vi "IMU State Machine.vi"(0 "error in":errorcluster, 11 "IMU Command":T1) -> (2 "Gyro xyz (rad/s)":dbl[](array[numeric]), 3 "Acceleration x,y,z":dbl[](array[numeric]), 8 "error out":errorcluster)   [LabVIEW 2016]
uses:
  IMU Cmd.ctl
panel:
  out "Gyro x,y,z (deg/s)":dbl[](array[numeric])
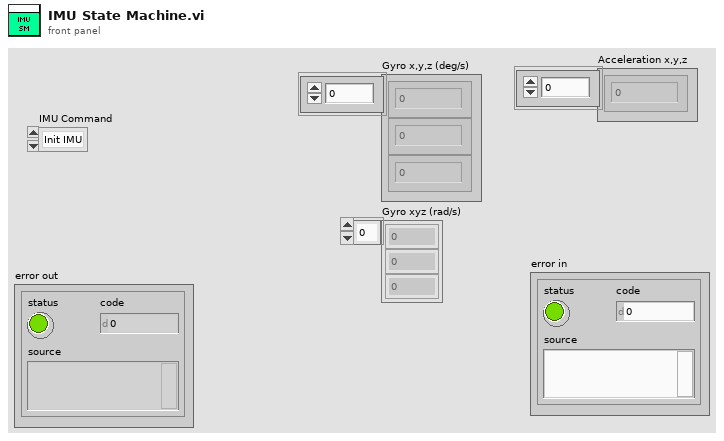
[diagram p1: front panel]
types:
  T1 = typedef "IMU Cmd.ctl" = enum16{"Init IMU", "Calibrate", "Read motion"}
  T2 = typedef "I2C.lvlib/I2C Reference.ctl" = cluster{"myRIO Reference":T3, "I2C Channels Enum":T7, "I2C Configuration":T8}
  T3 = typedef "myRIO Generic Hardware Reference.ctl" = cluster{"myRIO Model":T4, "myRIO Hardware Reference":T5}
  T4 = typedef "Hardware Version Enum.ctl" = enum16{"Unknown", "myRIO-1900", "myRIO-1950", "roboRIO", "NI ELVIS RIO CM"}
  T5 = typedef "myRIO v1.0 Reference.ctl" = cluster{"Generic FPGA Reference":T6, "Allow multiple opens":bool}
  T6 = typedef "Generic FPGA Reference.ctl" = refnum<k20>
  T7 = typedef "I2C Channels Enum.ctl" = enum16{"Not Connected", "A/I2C", "B/I2C", "I2C/I2C"}
  T8 = typedef "I2C.lvlib/I2C Configuration.ctl" = cluster{"I2C Transfer Rate":T9}
  T9 = typedef "I2C.lvlib/I2C Transfer Rate.ctl" = enum16{"Standard mode (100 kbps)", "Fast mode (400 kbps)"}
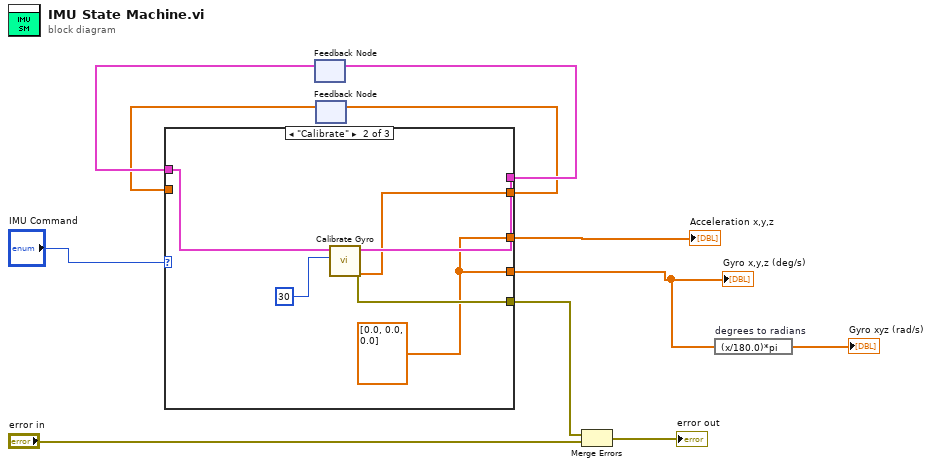
[diagram p0: block diagram]
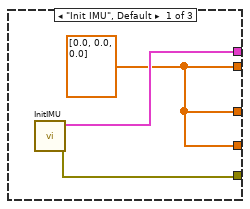
[diagram p2: hidden frame]
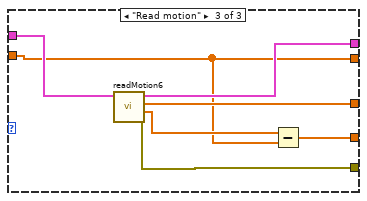
[diagram p3: hidden frame]
diagram:
  n1 = feedback #1() -> (w6:T2)  [unwired: 1 in]
  n2 = feedback #2() -> (w4:dbl[])  [unwired: 1 in]
  n3 = case shown="\"Calibrate\"" "IMU Command" {
    tunnel: [w14 w16 w26] -> w8
    tunnel: [w13 w19 w25] -> w7
    tunnel: w6 -> [_ w20 w27]
    tunnel: [w12 w18 w22] -> w5
    tunnel: w4 -> [_ _ w22]
    tunnel: [w12 w15 w24] -> w3
    tunnel: [w12 w15 w21] -> w2
    frame "Init IMU", Default {
      w12 = dbl[] [0.0, 0.0, 0.0] ("Bias Gyro")
      n4 = call "InitIMU.vi"() -> ("error out"=w14:errorcluster, "I2C Ref Out"=w13:T2)  [unwired: 10 in]
    }
    frame "Calibrate" {
      w15 = dbl[] [0.0, 0.0, 0.0] ("Acceleration x,y,z")
      n5 = call "Calibrate Gyro.vi"("Times"=30, "I2C Ref In"=w20) -> ("error out"=w16:errorcluster, "Bias Gyro"=w18:dbl[], "I2C Ref Out"=w19:T2)  [unwired: 7 in]
    }
    frame "Read motion" {
      n6 = call "readMotion6.vi"("I2C Ref Out"=w27) -> ("error out"=w26:errorcluster, "Gyro x,y,z (deg/s)"=w23:dbl[], "Acceleration x,y,z"=w24:dbl[], "I2C Ref Out 2"=w25:T2)  [unwired: 7 in]
      n7 = Subtract(x=w23, y=w22) -> (x-y=w21:dbl[])
    }
  }
  "Acceleration x,y,z" <- w3
  "Gyro x,y,z (deg/s)" <- w2
  n8 = feedback-in #1(w7) -> ()
  n9 = feedback-in #2(w5) -> ()
  n10 = Merge Errors(w8, "error in") -> (→"error out":errorcluster)
  n11 = expression code="(x/180.0)*pi" "degrees to radians"(w2) -> (→"Gyro xyz (rad/s)":dbl[])
